vi "S2C_VLFT10_Proc_FirstBootAlarms.vi"(8 "Error In":errorcluster, 11 "Exceptions":string) -> (0 "Error Out":errorcluster, 3 "Pass?":string)   [LabVIEW 2015]
uses:
  Fornax/VIs/S2C_FORNAX_Proc_Globals.vi
  XML/S2C_XML_Globals.vi
  <vilib>/regexp/Match Regular Expression.xnode
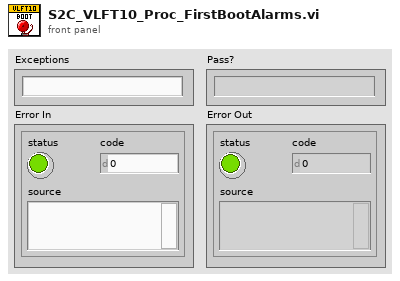
[diagram p1: front panel]
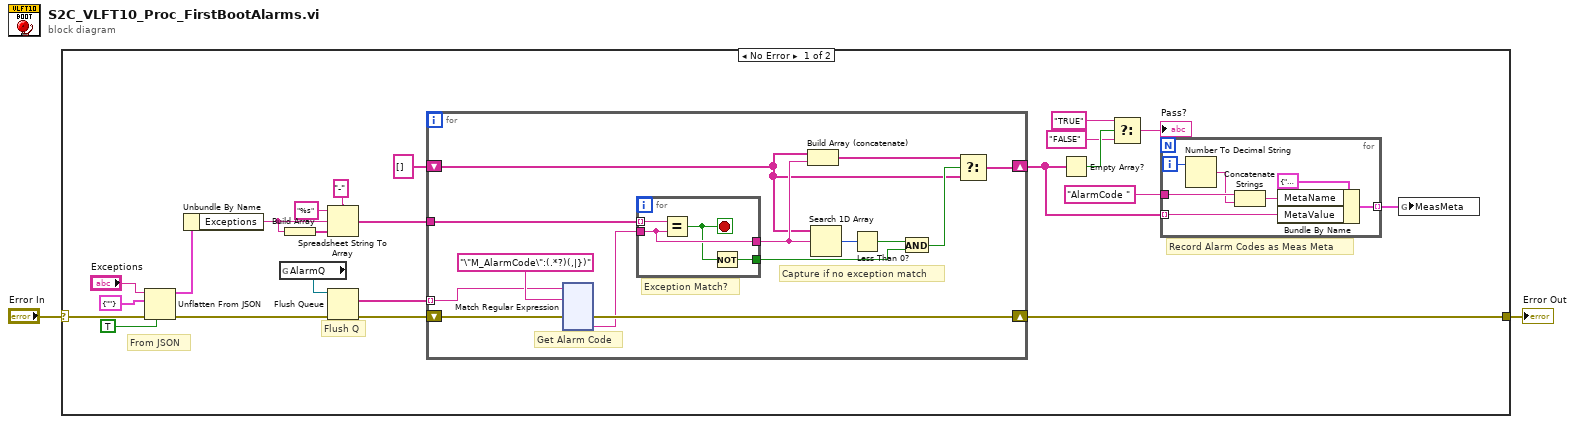
[diagram p0: block diagram]
diagram:
  n1 = case shown="No Error" "Error In" {
    selector: "Error In" -> [w10 w167]
    tunnel: [w22 w167] -> w1
    frame No Error {
      # "Flush Q"
      # "From JSON"
      # "Record Alarm Codes as Meas Meta"
      n2 = Unflatten From JSON(JSON string="Exceptions", type and defaults=cluster{"Exceptions":string} {"Exceptions"=""}, default null elements? (F)=TRUE, error in (no error)=w10) -> (value=w6:cluster{"Exceptions":string}, error out=w4:errorcluster)  [unwired: 3 in]
      n3 = Unbundle By Name(w6) -> ("Exceptions"=w5:string)
      n4 = global read "S2C_FORNAX_Proc_Globals.vi" "AlarmQ"() -> (w3:refnum<queue>)
      n5 = Build Array(w5) -> (w25:string[])
      n6 = Spreadsheet String To Array(delimiter (Tab)="-", format string="%s", spreadsheet string=w5, array type (2D Dbl)=w25) -> (array=w19:string[])
      n7 = Flush Queue(queue=w3, error in (no error)=w4) -> (remaining elements=w20:string[], error out=w21:errorcluster)  [unwired: 1 out]
      n8 = for {
        tunnel: w20 -> [w43] mode=indexing
        tunnel: w19 -> [w42]
        shift-right: [w38] -> w17
        shift-left: string[] [] -> [w33]
        shift-right: [w45] -> w22
        shift-left: w21 -> [w44]
        # "Capture if no exception match"
        # "Exception Match?"
        # "Get Alarm Code"
        n9 = xnode "Match Regular Expression"("input string"=w43, "regular expression"="\"M_AlarmCode\":(.*?)(,|})" ("format string"), "error in"=w44) -> ("error out"=w45:errorcluster, "submatch 1"=w41:string)  [unwired: 3 in, 4 out]
        n10 = for {
          tunnel: w42 -> [w50] mode=indexing
          tunnel: w41 -> [w49]
          tunnel: [w49] -> w39
          tunnel: [w47] -> w37
          stop <- w48 stop-if-true
          n11 = Equal?(x=w50, y=w49) -> (x = y?=w48:bool)
          n12 = Not(x=w48) -> (.not. x?=w47:bool)
        }
        n13 = Build Array (concatenate)(w33, w39) -> (w34:string[])
        n14 = Search 1D Array(1D array=w33, element=w39) -> (index of element=w40:i32)  [unwired: 1 in]
        n15 = Less Than 0?(x=w40) -> (x < 0?=w36:bool)
        n16 = And(x=w36, y=w37) -> (x .and. y?=w35:bool)
        n17 = Select(t=w34, s=w35, f=w33) -> (s? t:f=w38:string[])
      }
      n18 = Empty Array?(array=w17) -> (empty?=w14:bool)
      n19 = Select(t="TRUE", s=w14, f="FALSE") -> (s? t:f=→"Pass?":string)
      n20 = for {
        tunnel: w17 -> [w27] mode=indexing
        tunnel: "AlarmCode " -> [w30]
        tunnel: [w26] -> w15 mode=indexing
        i -> [w31]
        n21 = Number To Decimal String(number=w31) -> (decimal integer string=w29:string)  [unwired: 1 in]
        n22 = Concatenate Strings(w30, w29) -> (w28:string)
        n23 = Bundle By Name(cluster=cluster{"MetaName":string, "MetaValue":string} {"MetaName"="", "MetaValue"=""}, "MetaName"=w28, "MetaValue"=w27) -> (w26:cluster{"MetaName":string, "MetaValue":string})
      }
      n24 = global write "S2C_XML_Globals.vi" "MeasMeta"(w15) -> ()
    }
    frame Error {
    }
  }
  "Error Out" <- w1
